vi "Simulated_Field_FIELD_ODOM_CLAMP.vi"(9 "Robot Half Width M":dbl, 10 "Robot Half Length M":dbl, 11 "in Sim Pose":T1={"TRANSLATION"={"X"=0.0, "Y"=0.0}, "ROTATION"={"VALUE"=0.0, "COS"=1.0, "SIN"=0.0}} {"ROTATION"."SIN" format="%13.4f"; "ROTATION"."COS" format="%13.4f"; "ROTATION"."VALUE" format="%13.4f"; "TRANSLATION"."Y" format="%14.3f"; "TRANSLATION"."X" format="%14.3f"}) -> (3 "out Sim Pose":T1={"TRANSLATION"={"X"=0.0, "Y"=0.0}, "ROTATION"={"VALUE"=0.0, "COS"=1.0, "SIN"=0.0}} {"ROTATION"."SIN" format="%13.4f"; "ROTATION"."COS" format="%13.4f"; "ROTATION"."VALUE" format="%13.4f"; "TRANSLATION"."Y" format="%14.3f"; "TRANSLATION"."X" format="%14.3f"})   [LabVIEW 2019, in "Simulated_Field.lvlib"]
uses:
  Simulated_Field.lvlib
  <vilib>/Rock Robotics/WPI/ThirdParty/JAS_Junk/TrajLib/TypeDef/POSE2D.ctl
  <vilib>/Rock Robotics/WPI/ThirdParty/JAS_Junk/TrajLib/TypeDef/TRANSLATION2D.ctl
  <vilib>/Rock Robotics/WPI/ThirdParty/JAS_Junk/TrajLib/TypeDef/ROTATION2D.ctl
  <vilib>/Rock Robotics/WPI/ThirdParty/JAS_Junk/TrajLib/Trajectory_Library.lvlib
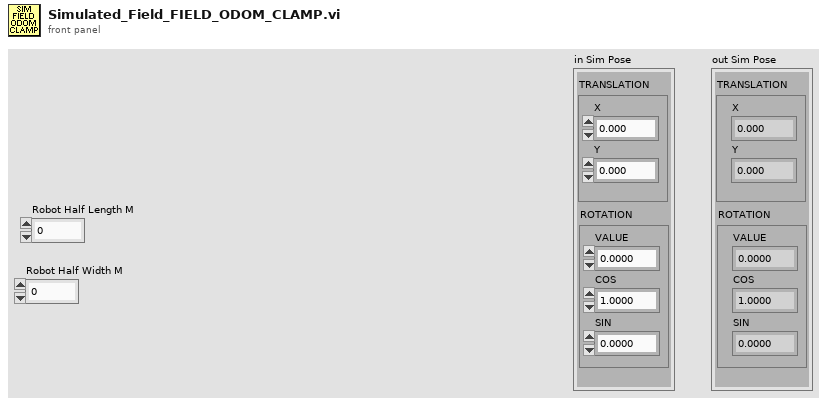
[diagram p1: front panel]
types:
  T1 = typedef "Trajectory_Library.lvlib/POSE2D.ctl" = cluster{"TRANSLATION":T2, "ROTATION":T3}
  T2 = typedef "Trajectory_Library.lvlib/TRANSLATION2D.ctl" = cluster{"X":dbl, "Y":dbl}
  T3 = typedef "Trajectory_Library.lvlib/ROTATION2D.ctl" = cluster{"VALUE":dbl, "COS":dbl, "SIN":dbl}
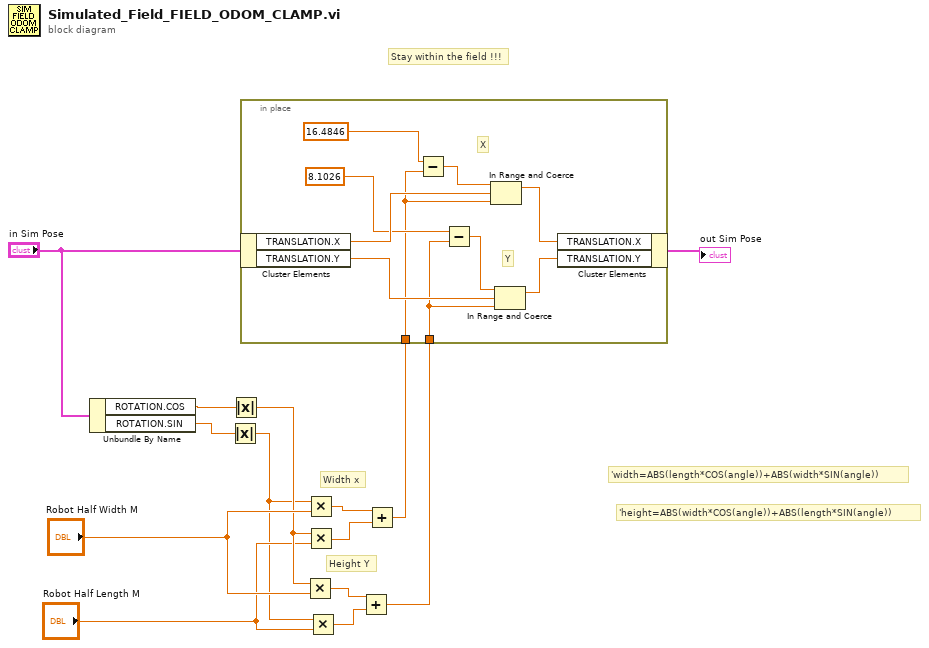
[diagram p0: block diagram]
diagram:
  # "'width=ABS(length*COS(angle))+ABS(width*SIN(angle))"
  # "Height Y"
  # "Width x"
  # "'height=ABS(width*COS(angle))+ABS(length*SIN(angle))"
  # "Stay within the field !!!"
  n1 = Unbundle By Name("in Sim Pose") -> ("ROTATION.COS"=w12:dbl, "ROTATION.SIN"=w11:dbl)
  n2 = Absolute Value(x=w11) -> (abs(x)=w1:dbl)
  n3 = Absolute Value(x=w12) -> (abs(x)=w3:dbl)
  n4 = Multiply(x=w3, y="Robot Half Width M") -> (x*y=w7:dbl)
  n5 = Multiply(x=w1, y="Robot Half Width M") -> (x*y=w10:dbl)
  n6 = Multiply(x=w3, y="Robot Half Length M") -> (x*y=w9:dbl)
  n7 = Multiply(x=w1, y="Robot Half Length M") -> (x*y=w6:dbl)
  n8 = Add(x=w7, y=w6) -> (x+y=w5:dbl)
  n9 = Add(x=w10, y=w9) -> (x+y=w8:dbl)
  n10 = in-place {
    in-place-border: w8 -> [w16]
    in-place-border: w5 -> [w15]
    # "Y"
    # "X"
    n11 = in-place-cluster #1("in Sim Pose") -> ("TRANSLATION.X"=w22:dbl, "TRANSLATION.Y"=w23:dbl)
    n12 = Subtract(x=16.4846 ("upper limit"), y=w16) -> (x-y=w19:dbl)
    n13 = Subtract(x=8.1026 ("upper limit"), y=w15) -> (x-y=w17:dbl)
    n14 = In Range and Coerce(upper limit=w19, x=w22, lower limit=w16) -> (coerced(x)=w24:dbl)  [unwired: 1 out]
    n15 = In Range and Coerce(upper limit=w17, x=w23, lower limit=w15) -> (coerced(x)=w21:dbl)  [unwired: 1 out]
    n16 = in-place-cluster #1("TRANSLATION.X"=w24, "TRANSLATION.Y"=w21) -> (→"out Sim Pose":T1)
  }
